vi "Read.vi"(8 "error in (no error)":errorcluster, 11 "Honeywell Compass HMC6343":refnum<class "Honeywell Compass HMC6343.lvclass">) -> (0 "error out":errorcluster, 2 "Data":T1, 3 "Honeywell Compass HMC6343 out":refnum<class "Honeywell Compass HMC6343.lvclass">)   [LabVIEW 2019, in "Honeywell Compass HMC6343.lvclass"]
doc: "Reads the Acceleration, Magnetic Field, Heading and Tilt Data."
uses:
  Honeywell Compass HMC6343.lvclass
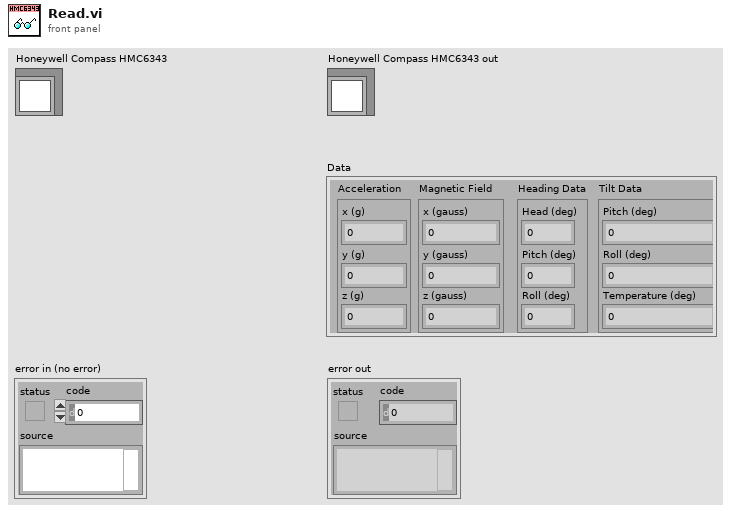
[diagram p1: front panel]
types:
  T1 = cluster{"Acceleration":cluster{"x (g)":dbl, "y (g)":dbl, "z (g)":dbl}, "Magnetic Field":cluster{"x (gauss)":dbl, "y (gauss)":dbl, "z (gauss)":dbl}, "Heading Data":cluster{"Head (deg)":dbl, "Pitch (deg)":dbl, "Roll (deg)":dbl}, "Tilt Data":cluster{"Pitch (deg)":dbl, "Roll (deg)":dbl, "Temperature (deg)":dbl}}
  T2 = cluster{"x (gauss)":dbl, "y (gauss)":dbl, "z (gauss)":dbl}
  T3 = cluster{"Head (deg)":dbl, "Pitch (deg)":dbl, "Roll (deg)":dbl}
  T4 = cluster{"Pitch (deg)":dbl, "Roll (deg)":dbl, "Temp (deg)":dbl}
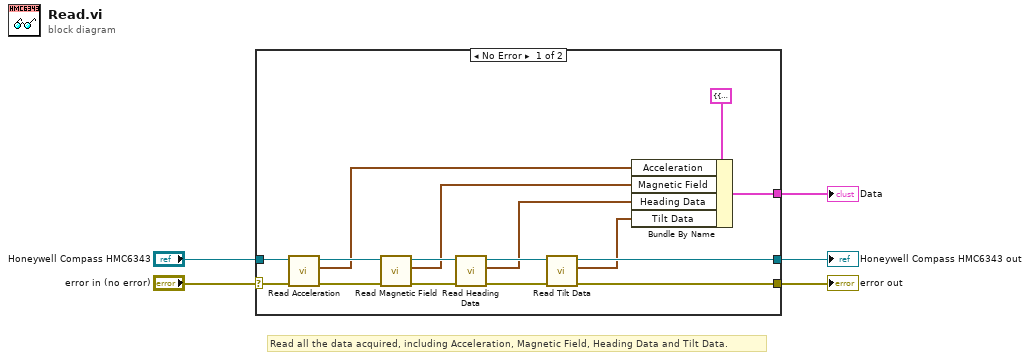
[diagram p0: block diagram]
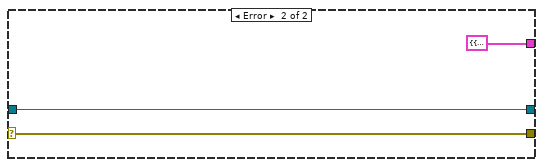
[diagram p2: hidden frame]
diagram:
  # "Read all the data acquired, including Acceleration, Magnetic Field, Heading Data and Tilt Data."
  n1 = case shown="No Error" "error in (no error)" {
    selector: "error in (no error)" -> [w16 w24]
    tunnel: "Honeywell Compass HMC6343" -> [w21 w23]
    tunnel: [w17 w23] -> w4
    tunnel: [w12 w24] -> w2
    tunnel: [w6 T1 {"Acceleration"={"x (g)"=0.0, "y (g)"=0.0, "z (g)"=0.0}, "Magnetic Field"={"x (gauss)"=0.0, "y (gauss)"=0.0, "z (gauss)"=0.0}, "Heading Data"={"Head (deg)"=0.0, "Pitch (deg)"=0.0, "Roll (deg)"=0.0}, "Tilt Data"={"Pitch (deg)"=0.0, "Roll (deg)"=0.0, "Temperature (deg)"=0.0}} ("output data cluster")] -> w1
    frame No Error {
      n2 = call-dynamic "Read Acceleration.vi"("error in (no error)"=w16, "Honeywell Compass HMC6343"=w21) -> ("error out"=w15:errorcluster, "Acceleration"=w10:cluster{"x (g)":dbl, "y (g)":dbl, "z (g)":dbl}, "Honeywell Compass HMC6343 out"=w20:refnum<class "Honeywell Compass HMC6343.lvclass">)  [unwired: 7 in]
      n3 = call-dynamic "Read Magnetic Field.vi"("error in (no error)"=w15, "Honeywell Compass HMC6343"=w20) -> ("error out"=w14:errorcluster, "Magnetic Field"=w9:T2, "Honeywell Compass HMC6343 out"=w19:refnum<class "Honeywell Compass HMC6343.lvclass">)  [unwired: 7 in]
      n4 = call-dynamic "Read Heading Data.vi"("error in (no error)"=w14, "Honeywell Compass HMC6343"=w19) -> ("error out"=w13:errorcluster, "Heading Data"=w8:T3, "Honeywell Compass HMC6343 out"=w18:refnum<class "Honeywell Compass HMC6343.lvclass">)  [unwired: 7 in]
      n5 = call-dynamic "Read Tilt Data.vi"("error in (no error)"=w13, "Honeywell Compass HMC6343"=w18) -> ("error out"=w12:errorcluster, "Tilt Data"=w7:T4, "Honeywell Compass HMC6343 out"=w17:refnum<class "Honeywell Compass HMC6343.lvclass">)  [unwired: 7 in]
      n6 = Bundle By Name(cluster=T1 {"Acceleration"={"x (g)"=0.0, "y (g)"=0.0, "z (g)"=0.0}, "Magnetic Field"={"x (gauss)"=0.0, "y (gauss)"=0.0, "z (gauss)"=0.0}, "Heading Data"={"Head (deg)"=0.0, "Pitch (deg)"=0.0, "Roll (deg)"=0.0}, "Tilt Data"={"Pitch (deg)"=0.0, "Roll (deg)"=0.0, "Temperature (deg)"=0.0}} ("output data cluster"), "Acceleration"=w10, "Magnetic Field"=w9, "Heading Data"=w8, "Tilt Data"=w7) -> (w6:T1)
    }
    frame Error {
    }
  }
  "error out" <- w2
  "Honeywell Compass HMC6343 out" <- w4
  "Data" <- w1
